vi "000TemplateCommand.vi"(7 "Parameters":dbl[](array[numeric]), 11 "Startup":bool) -> (4 "Completed":bool, 15 "Reinit":bool)   [LabVIEW 2019]
uses:
  Auto Utilities/Command_Execution_State.ctl
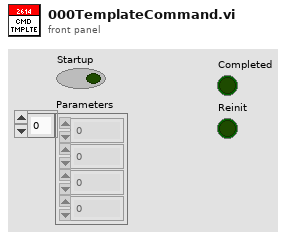
[diagram p1: front panel]
types:
  T1 = typedef "Command_Execution_State.ctl" = enum16{"Initialize", "Execute", "Finish"}
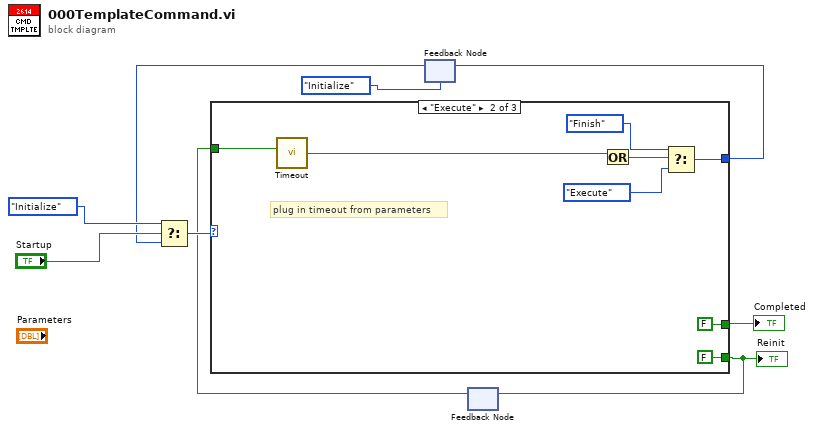
[diagram p0: block diagram]
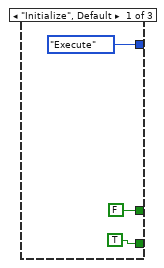
[diagram p2: hidden frame]
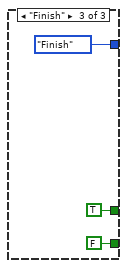
[diagram p3: hidden frame]
diagram:
  n1 = feedback #1(Command_Execution_State."Initialize") -> (w5:T1)
  n2 = Select(t=Command_Execution_State."Initialize", s="Startup", f=w5) -> (s? t:f=w7:T1)
  n3 = feedback #2() -> (w1:bool)  [unwired: 1 in]
  n4 = case shown="\"Execute\"" w7 {
    tunnel: [Command_Execution_State."Execute" w18 Command_Execution_State."Finish"] -> w6
    tunnel: [FALSE ("Reinit") FALSE ("Reinit") TRUE ("Reinit")] -> w3
    tunnel: [TRUE ("Reinit") FALSE ("Reinit") FALSE ("Reinit")] -> w2
    tunnel: w1 -> [_ w15 _]
    frame "Initialize", Default {
    }
    frame "Execute" {
      # "plug in timeout from parameters"
      n5 = call "Timeout.vi"("Initialize"=w15) -> ("Timed Out?"=w13:bool)  [unwired: 1 in]
      n6 = Or(x=w13) -> (x .or. y?=w14:bool)  [unwired: 1 in]
      n7 = Select(t=Command_Execution_State."Finish", s=w14, f=Command_Execution_State."Execute") -> (s? t:f=w18:T1)
    }
    frame "Finish" {
    }
  }
  "Reinit" <- w2
  "Completed" <- w3
  n8 = feedback-in #1(w6) -> ()
  n9 = feedback-in #2(w2) -> ()
